vi "Feng.vi"(2 "decimal 2":i32) -> (0 "bitstream 3":i32[](array[numeric]))   [LabVIEW 2020]
panel:
  out "Numeric":i32
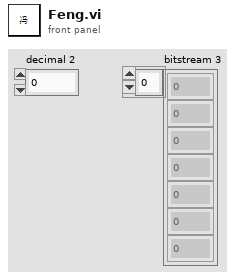
[diagram p1: front panel]
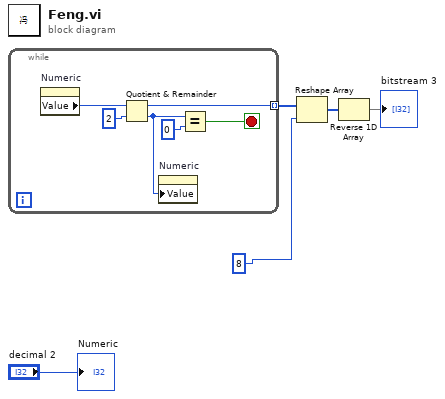
[diagram p0: block diagram]
diagram:
  n1 = while {
    tunnel: [w10] -> w3 mode=indexing
    stop <- w9 stop-if-true
    n2 = property on="Numeric" class="DigNum (strict)"() -> ("Value"=w7:i32)  [unwired: 2 in, 2 out]
    n3 = Quotient & Remainder(x=w7, y=2) -> (x-y*floor(x/y)=w10:i32, floor(x/y)=w6:i32)
    n4 = property on="Numeric" class="DigNum (strict)"("Value"=w6) -> ()  [unwired: 2 in, 2 out]
    n5 = Equal?(x=w6, y=0) -> (x = y?=w9:bool)
  }
  n6 = Reshape Array(w3, 8 ("dimension size")) -> (w5:i32[])
  n7 = Reverse 1D Array(array=w5) -> (reversed array=→"bitstream 3":i32[])
  "Numeric" <- "decimal 2"
